vi "Build.vi"(0 "version":string, 1 "Progress Bar":refnum<vi>, 5 "iss path":string) -> ()   [LabVIEW 2020]
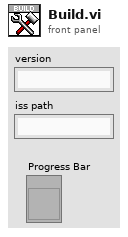
[diagram p1: front panel]
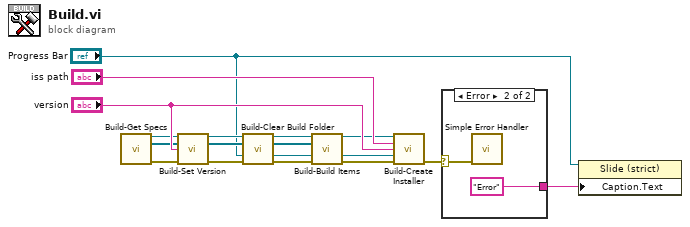
[diagram p0: block diagram]
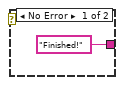
[diagram p2: hidden frame]
diagram:
  n1 = call "Build-Get Specs.vi"() -> ("project"=w15:refnum<vi>, "specs"=w14:refnum<vi>[], "error out"=w16:errorcluster)  [unwired: 13 in]
  n2 = call "Build-Set Version.vi"("project"=w15, "specs"=w14, "Version"="version", "error in (no error)"=w16) -> ("project out"=w11:refnum<vi>, "specs thru"=w12:refnum<vi>[], "error out"=w13:errorcluster)  [unwired: 9 in]
  n3 = call "Build-Clear Build Folder.vi"("project in"=w11, "specs in"=w12, "slide in"="Progress Bar", "error in (no error)"=w13) -> ("project out"=w2:refnum<vi>, "specs thru"=w1:refnum<vi>[], "slide out"=w4:refnum<vi>, "error out"=w3:errorcluster)  [unwired: 8 in]
  n4 = call "Build-Build Items.vi"("project in"=w2, "specs in"=w1, "slide in"=w4, "error in (no error)"=w3) -> ("project out"=w8:refnum<vi>, "slide out"=w9:refnum<vi>, "error out"=w7:errorcluster)  [unwired: 9 in]
  n5 = call "Build-Create Installer.vi"("project in"=w8, "iss name"="iss path", "version"="version", "slide in"=w9, "error in (no error)"=w7) -> ("error out"=w6:errorcluster)  [unwired: 10 in]
  n6 = case shown="Error" w6 {
    selector: w6 -> [_ w20]
    tunnel: ["Finished!" "Error"] -> w5
    frame No Error {
    }
    frame Error {
      n7 = call <vilib>:"Simple Error Handler.vi"("error in (no error)"=w20) -> ()  [unwired: 4 in, 5 out]
    }
  }
  n8 = property on="Property Node" class="Slide (strict)"(reference="Progress Bar", "Caption.Text"=w5) -> ()  [unwired: 1 in, 2 out]
